vi "输入数据解析.vi"(0 "单个参数补充":dbl, 1 "从板号":dbl=1.0, 2 "主板二维码":string="BNET01", 3 "从板二维码":string="BNET01", 5 "主板引用":refnum<vi>, 7 "从板引用":refnum<vi>, 9 "主板选项":string="三级故障阀值", 11 "枚举":enum16{"主板", "从板"}(ring), 12 "快换":bool caption="快换写入") -> (4 "输出数组":dbl[][](array[numeric]), 6 "数组长度":dbl[](array[numeric]), 8 "循环次数":i32, 10 "命令":u32, 14 "名称":string[](array[string]), 15 "命令序号":u32[](array[numeric]))   [LabVIEW 2013] (continued)
                  disable-tunnel: [w17680 w17684] -> w17676
                  disable-tunnel: w17674 -> [w17679 _]
                  frame Disabled {
                    n6928 = Unbundle By Name(w17679) -> ("电压过高"=w17678:dbl)
                    n6929 = call "输入分辨率计算-EV05.vi"("1字节?"=FALSE, "数值"=w17678, "分辨率"=0.1) -> ("低字节"=w17680:dbl, "高字节1"=w17681:dbl)  [unwired: 2 in, 5 out]
                  }
                  frame Enabled {
                    w17684 = 255 ("高字节1")
                  }
                }
                n6930 = Build Array(w17677, w17676) -> (w17675:i32[])
              }
              frame 1 {
                # "电压过低"
                n6931 = disable-structure shown="启用" {
                  disable-tunnel: [w17692 w17695] -> w17688
                  disable-tunnel: [w17691 w17695] -> w17687
                  disable-tunnel: w17685 -> [w17690 _]
                  frame Disabled {
                    n6932 = Unbundle By Name(w17690) -> ("电压过低"=w17689:dbl)
                    n6933 = call "输入分辨率计算-EV05.vi"("1字节?"=FALSE, "数值"=w17689, "分辨率"=0.1) -> ("低字节"=w17691:dbl, "高字节1"=w17692:dbl)  [unwired: 2 in, 5 out]
                  }
                  frame Enabled {
                    w17695 = 255 ("高字节1")
                  }
                }
                n6934 = Build Array(w17688, w17687) -> (w17686:i32[])
              }
              frame 2 {
                # "电压不均衡"
                n6935 = disable-structure shown="启用" {
                  disable-tunnel: [w17703 w17706] -> w17699
                  disable-tunnel: [w17702 w17706] -> w17698
                  disable-tunnel: w17696 -> [w17701 _]
                  frame Disabled {
                    n6936 = Unbundle By Name(w17701) -> ("电压不均衡(V)"=w17700:dbl)
                    n6937 = call "输入分辨率计算-EV05.vi"("1字节?"=FALSE, "数值"=w17700, "分辨率"=0.1) -> ("低字节"=w17702:dbl, "高字节1"=w17703:dbl)  [unwired: 2 in, 5 out]
                  }
                  frame Enabled {
                    w17706 = 255 ("高字节1")
                  }
                }
                n6938 = Build Array(w17699, w17698) -> (w17697:i32[])
              }
              frame 3 {
                # "温度过高"
                n6939 = disable-structure shown="启用" {
                  disable-tunnel: [w17713 255 ("高字节1")] -> w17709
                  disable-tunnel: w17707 -> [w17711 _]
                  frame Enabled {
                    n6940 = Unbundle By Name(w17711) -> ("温度过高"=w17710:dbl)
                    n6941 = call "输入分辨率计算-EV05.vi"("1字节?"=TRUE, "数值"=w17710, "偏移量"=-40.0, "分辨率"=1.0) -> ("高字节1"=w17713:dbl)  [unwired: 1 in, 6 out]
                  }
                  frame Disabled {
                  }
                }
                n6942 = Build Array(w17709) -> (w17708:dbl[])
              }
              frame 4 {
                # "温度过低"
                n6943 = disable-structure shown="启用" {
                  disable-tunnel: [w17723 255 ("高字节1")] -> w17719
                  disable-tunnel: w17717 -> [w17721 _]
                  frame Disabled {
                    n6944 = Unbundle By Name(w17721) -> ("温度过低"=w17720:dbl)
                    n6945 = call "输入分辨率计算-EV05.vi"("1字节?"=TRUE, "数值"=w17720, "偏移量"=-40.0, "分辨率"=1.0) -> ("高字节1"=w17723:dbl)  [unwired: 1 in, 6 out]
                  }
                  frame Enabled {
                  }
                }
                n6946 = Build Array(w17719) -> (w17718:i32[])
              }
              frame 5 {
                # "温度不均衡"
                n6947 = disable-structure shown="启用" {
                  disable-tunnel: [w17732 255 ("高字节1")] -> w17729
                  disable-tunnel: w17727 -> [w17731 _]
                  frame Disabled {
                    n6948 = Unbundle By Name(w17731) -> ("温度不均衡"=w17730:dbl)
                    n6949 = call "输入分辨率计算-EV05.vi"("1字节?"=TRUE, "数值"=w17730, "分辨率"=1.0) -> ("高字节1"=w17732:dbl)  [unwired: 2 in, 6 out]
                  }
                  frame Enabled {
                  }
                }
                n6950 = Build Array(w17729) -> (w17728:i32[])
              }
              frame 6 {
                # "SOC过低"
                n6951 = disable-structure shown="启用" {
                  disable-tunnel: w17738 -> [w17755 _]
                  disable-tunnel: [w17741 w17758] -> w17737
                  disable-tunnel: [w17740 w17758] -> w17736
                  frame Disabled {
                    n6952 = Unbundle By Name(w17755) -> ("SOC过低"=w17754:dbl)
                    n6953 = call "输入分辨率计算-EV05.vi"("1字节?"=FALSE, "数值"=w17754, "分辨率"=0.1) -> ("低字节"=w17743:dbl, "高字节1"=w17744:dbl)  [unwired: 2 in, 5 out]
                    n6954 = call "二进制解析-8.6.vi"("索引"=4, "数值"=0) -> ("低位子数组"=w17747:i32[])  [unwired: 3 out]
                    n6955 = call "二进制解析-8.6.vi"("索引"=4, "数值"=w17744) -> ("低位子数组"=w17750:i32[])  [unwired: 3 out]
                    n6956 = call "二进制解析-8.6.vi"("索引"=4, "数值"=w17743) -> ("低位子数组"=w17748:i32[], "高位子数组"=w17749:i32[])  [unwired: 2 out]
                    n6957 = Insert Into Array(array=w17750, new element=w17749) -> (w17752:i32[])  [unwired: 1 in]
                    n6958 = Insert Into Array(array=w17748, new element=w17747) -> (w17746:i32[])  [unwired: 1 in]
                    n6959 = call "数值二进制转十进制-8.6.vi"("子数组"=w17746) -> ("十进制数值"=w17741:i32)  [unwired: 4 out]
                    n6960 = call "数值二进制转十进制-8.6.vi"("子数组"=w17752) -> ("十进制数值"=w17740:i32)  [unwired: 4 out]
                  }
                  frame Enabled {
                    w17758 = 255 ("高字节1")
                  }
                }
                n6961 = Build Array(w17736, w17737) -> (w17739:i32[])
              }
            }
            n6962 = Insert Into Array(array=w17670, new element=w17669) -> (w17671:dbl[])  [unwired: 1 in]
          }
          n6963 = Build Array(w17664) -> (w17663:dbl[][])
        }
        frame "温度过高(3)" {
          n6964 = Unbundle By Name(w17763) -> ("三级故障(从板)"=w17764:refnum<vi>)
          n6965 = property class="Clust (严格)"(reference=w17764) -> ("Value"=w17762:T8)  [unwired: 1 in, 2 out]
          n6966 = for {
            N: 7 -> [_]
            tunnel: w17762 -> [w17774]
            shift-right: [w17773] -> w17766
            shift-left: dbl[] [] -> [w17772]
            i -> [w17775]
            n6967 = case shown="3" w17775 {
              tunnel: w17774 -> [w17776 w17787 w17798 w17809 w17819 w17829 w17840]
              tunnel: [w17777 w17788 w17799 w17810 w17820 w17830 w17841] -> w17771
              frame 0, Default {
                # "电压过高"
                n6968 = disable-structure shown="启用" {
                  disable-tunnel: [w17783 w17786] -> w17779
                  disable-tunnel: [w17782 w17786] -> w17778
                  disable-tunnel: w17776 -> [w17781 _]
                  frame Disabled {
                    n6969 = Unbundle By Name(w17781) -> ("电压过高"=w17780:dbl)
                    n6970 = call "输入分辨率计算-EV05.vi"("1字节?"=FALSE, "数值"=w17780, "分辨率"=0.1) -> ("低字节"=w17782:dbl, "高字节1"=w17783:dbl)  [unwired: 2 in, 5 out]
                  }
                  frame Enabled {
                    w17786 = 255 ("高字节1")
                  }
                }
                n6971 = Build Array(w17779, w17778) -> (w17777:i32[])
              }
              frame 1 {
                # "电压过低"
                n6972 = disable-structure shown="启用" {
                  disable-tunnel: [w17794 w17797] -> w17790
                  disable-tunnel: [w17793 w17797] -> w17789
                  disable-tunnel: w17787 -> [w17792 _]
                  frame Disabled {
                    n6973 = Unbundle By Name(w17792) -> ("电压过低"=w17791:dbl)
                    n6974 = call "输入分辨率计算-EV05.vi"("1字节?"=FALSE, "数值"=w17791, "分辨率"=0.1) -> ("低字节"=w17793:dbl, "高字节1"=w17794:dbl)  [unwired: 2 in, 5 out]
                  }
                  frame Enabled {
                    w17797 = 255 ("高字节1")
                  }
                }
                n6975 = Build Array(w17790, w17789) -> (w17788:i32[])
              }
              frame 2 {
                # "电压不均衡"
                n6976 = disable-structure shown="启用" {
                  disable-tunnel: [w17805 w17808] -> w17801
                  disable-tunnel: [w17804 w17808] -> w17800
                  disable-tunnel: w17798 -> [w17803 _]
                  frame Disabled {
                    n6977 = Unbundle By Name(w17803) -> ("电压不均衡(V)"=w17802:dbl)
                    n6978 = call "输入分辨率计算-EV05.vi"("1字节?"=FALSE, "数值"=w17802, "分辨率"=0.1) -> ("低字节"=w17804:dbl, "高字节1"=w17805:dbl)  [unwired: 2 in, 5 out]
                  }
                  frame Enabled {
                    w17808 = 255 ("高字节1")
                  }
                }
                n6979 = Build Array(w17801, w17800) -> (w17799:i32[])
              }
              frame 3 {
                # "温度过高"
                n6980 = disable-structure shown="启用" {
                  disable-tunnel: [w17815 255 ("高字节1")] -> w17811
                  disable-tunnel: w17809 -> [w17813 _]
                  frame Enabled {
                    n6981 = Unbundle By Name(w17813) -> ("温度过高"=w17812:dbl)
                    n6982 = call "输入分辨率计算-EV05.vi"("1字节?"=TRUE, "数值"=w17812, "偏移量"=-40.0, "分辨率"=1.0) -> ("高字节1"=w17815:dbl)  [unwired: 1 in, 6 out]
                  }
                  frame Disabled {
                  }
                }
                n6983 = Build Array(w17811) -> (w17810:dbl[])
              }
              frame 4 {
                # "温度过低"
                n6984 = disable-structure shown="启用" {
                  disable-tunnel: [w17825 255 ("高字节1")] -> w17821
                  disable-tunnel: w17819 -> [w17823 _]
                  frame Disabled {
                    n6985 = Unbundle By Name(w17823) -> ("温度过低"=w17822:dbl)
                    n6986 = call "输入分辨率计算-EV05.vi"("1字节?"=TRUE, "数值"=w17822, "偏移量"=-40.0, "分辨率"=1.0) -> ("高字节1"=w17825:dbl)  [unwired: 1 in, 6 out]
                  }
                  frame Enabled {
                  }
                }
                n6987 = Build Array(w17821) -> (w17820:i32[])
              }
              frame 5 {
                # "温度不均衡"
                n6988 = disable-structure shown="启用" {
                  disable-tunnel: [w17834 255 ("高字节1")] -> w17831
                  disable-tunnel: w17829 -> [w17833 _]
                  frame Disabled {
                    n6989 = Unbundle By Name(w17833) -> ("温度不均衡"=w17832:dbl)
                    n6990 = call "输入分辨率计算-EV05.vi"("1字节?"=TRUE, "数值"=w17832, "分辨率"=1.0) -> ("高字节1"=w17834:dbl)  [unwired: 2 in, 6 out]
                  }
                  frame Enabled {
                  }
                }
                n6991 = Build Array(w17831) -> (w17830:i32[])
              }
              frame 6 {
                # "SOC过低"
                n6992 = disable-structure shown="启用" {
                  disable-tunnel: w17840 -> [w17857 _]
                  disable-tunnel: [w17843 w17860] -> w17839
                  disable-tunnel: [w17842 w17860] -> w17838
                  frame Disabled {
                    n6993 = Unbundle By Name(w17857) -> ("SOC过低"=w17856:dbl)
                    n6994 = call "输入分辨率计算-EV05.vi"("1字节?"=FALSE, "数值"=w17856, "分辨率"=0.1) -> ("低字节"=w17845:dbl, "高字节1"=w17846:dbl)  [unwired: 2 in, 5 out]
                    n6995 = call "二进制解析-8.6.vi"("索引"=4, "数值"=0) -> ("低位子数组"=w17849:i32[])  [unwired: 3 out]
                    n6996 = call "二进制解析-8.6.vi"("索引"=4, "数值"=w17846) -> ("低位子数组"=w17852:i32[])  [unwired: 3 out]
                    n6997 = call "二进制解析-8.6.vi"("索引"=4, "数值"=w17845) -> ("低位子数组"=w17850:i32[], "高位子数组"=w17851:i32[])  [unwired: 2 out]
                    n6998 = Insert Into Array(array=w17852, new element=w17851) -> (w17854:i32[])  [unwired: 1 in]
                    n6999 = Insert Into Array(array=w17850, new element=w17849) -> (w17848:i32[])  [unwired: 1 in]
                    n7000 = call "数值二进制转十进制-8.6.vi"("子数组"=w17848) -> ("十进制数值"=w17843:i32)  [unwired: 4 out]
                    n7001 = call "数值二进制转十进制-8.6.vi"("子数组"=w17854) -> ("十进制数值"=w17842:i32)  [unwired: 4 out]
                  }
                  frame Enabled {
                    w17860 = 255 ("高字节1")
                  }
                }
                n7002 = Build Array(w17838, w17839) -> (w17841:i32[])
              }
            }
            n7003 = Insert Into Array(array=w17772, new element=w17771) -> (w17773:dbl[])  [unwired: 1 in]
          }
          n7004 = Build Array(w17766) -> (w17765:dbl[][])
        }
        frame "温度过低" {
          n7005 = Unbundle By Name(w17865) -> ("一级故障(从板)"=w17866:refnum<vi>)
          n7006 = property class="Clust (严格)"(reference=w17866) -> ("Value"=w17864:T8)  [unwired: 1 in, 2 out]
          n7007 = for {
            N: 7 -> [_]
            tunnel: w17864 -> [w17876]
            shift-right: [w17875] -> w17868
            shift-left: dbl[] [] -> [w17874]
            i -> [w17877]
            n7008 = case shown="4" w17877 {
              tunnel: w17876 -> [w17878 w17889 w17900 w17911 w17921 w17931 w17942]
              tunnel: [w17879 w17890 w17901 w17912 w17922 w17932 w17943] -> w17873
              frame 0, Default {
                # "电压过高"
                n7009 = disable-structure shown="启用" {
                  disable-tunnel: [w17885 w17888] -> w17881
                  disable-tunnel: [w17884 w17888] -> w17880
                  disable-tunnel: w17878 -> [w17883 _]
                  frame Disabled {
                    n7010 = Unbundle By Name(w17883) -> ("电压过高"=w17882:dbl)
                    n7011 = call "输入分辨率计算-EV05.vi"("1字节?"=FALSE, "数值"=w17882, "分辨率"=0.1) -> ("低字节"=w17884:dbl, "高字节1"=w17885:dbl)  [unwired: 2 in, 5 out]
                  }
                  frame Enabled {
                    w17888 = 255 ("高字节1")
                  }
                }
                n7012 = Build Array(w17881, w17880) -> (w17879:i32[])
              }
              frame 1 {
                # "电压过低"
                n7013 = disable-structure shown="启用" {
                  disable-tunnel: [w17896 w17899] -> w17892
                  disable-tunnel: [w17895 w17899] -> w17891
                  disable-tunnel: w17889 -> [w17894 _]
                  frame Disabled {
                    n7014 = Unbundle By Name(w17894) -> ("电压过低"=w17893:dbl)
                    n7015 = call "输入分辨率计算-EV05.vi"("1字节?"=FALSE, "数值"=w17893, "分辨率"=0.1) -> ("低字节"=w17895:dbl, "高字节1"=w17896:dbl)  [unwired: 2 in, 5 out]
                  }
                  frame Enabled {
                    w17899 = 255 ("高字节1")
                  }
                }
                n7016 = Build Array(w17892, w17891) -> (w17890:i32[])
              }
              frame 2 {
                # "电压不均衡"
                n7017 = disable-structure shown="启用" {
                  disable-tunnel: [w17907 w17910] -> w17903
                  disable-tunnel: [w17906 w17910] -> w17902
                  disable-tunnel: w17900 -> [w17905 _]
                  frame Disabled {
                    n7018 = Unbundle By Name(w17905) -> ("电压不均衡(V)"=w17904:dbl)
                    n7019 = call "输入分辨率计算-EV05.vi"("1字节?"=FALSE, "数值"=w17904, "分辨率"=0.1) -> ("低字节"=w17906:dbl, "高字节1"=w17907:dbl)  [unwired: 2 in, 5 out]
                  }
                  frame Enabled {
                    w17910 = 255 ("高字节1")
                  }
                }
                n7020 = Build Array(w17903, w17902) -> (w17901:i32[])
              }
              frame 3 {
                # "温度过高"
                n7021 = disable-structure shown="启用" {
                  disable-tunnel: [w17917 255 ("高字节1")] -> w17913
                  disable-tunnel: w17911 -> [w17915 _]
                  frame Disabled {
                    n7022 = Unbundle By Name(w17915) -> ("温度过高"=w17914:dbl)
                    n7023 = call "输入分辨率计算-EV05.vi"("1字节?"=TRUE, "数值"=w17914, "偏移量"=-40.0, "分辨率"=1.0) -> ("高字节1"=w17917:dbl)  [unwired: 1 in, 6 out]
                  }
                  frame Enabled {
                  }
                }
                n7024 = Build Array(w17913) -> (w17912:i32[])
              }
              frame 4 {
                # "温度过低"
                n7025 = disable-structure shown="启用" {
                  disable-tunnel: [w17927 255 ("高字节1")] -> w17923
                  disable-tunnel: w17921 -> [w17925 _]
                  frame Enabled {
                    n7026 = Unbundle By Name(w17925) -> ("温度过低"=w17924:dbl)
                    n7027 = call "输入分辨率计算-EV05.vi"("1字节?"=TRUE, "数值"=w17924, "偏移量"=-40.0, "分辨率"=1.0) -> ("高字节1"=w17927:dbl)  [unwired: 1 in, 6 out]
                  }
                  frame Disabled {
                  }
                }
                n7028 = Build Array(w17923) -> (w17922:dbl[])
              }
              frame 5 {
                # "温度不均衡"
                n7029 = disable-structure shown="启用" {
                  disable-tunnel: [w17936 255 ("高字节1")] -> w17933
                  disable-tunnel: w17931 -> [w17935 _]
                  frame Disabled {
                    n7030 = Unbundle By Name(w17935) -> ("温度不均衡"=w17934:dbl)
                    n7031 = call "输入分辨率计算-EV05.vi"("1字节?"=TRUE, "数值"=w17934, "分辨率"=1.0) -> ("高字节1"=w17936:dbl)  [unwired: 2 in, 6 out]
                  }
                  frame Enabled {
                  }
                }
                n7032 = Build Array(w17933) -> (w17932:i32[])
              }
              frame 6 {
                # "SOC过低"
                n7033 = disable-structure shown="启用" {
                  disable-tunnel: w17942 -> [w17959 _]
                  disable-tunnel: [w17945 w17962] -> w17941
                  disable-tunnel: [w17944 w17962] -> w17940
                  frame Disabled {
                    n7034 = Unbundle By Name(w17959) -> ("SOC过低"=w17958:dbl)
                    n7035 = call "输入分辨率计算-EV05.vi"("1字节?"=FALSE, "数值"=w17958, "分辨率"=0.1) -> ("低字节"=w17947:dbl, "高字节1"=w17948:dbl)  [unwired: 2 in, 5 out]
                    n7036 = call "二进制解析-8.6.vi"("索引"=4, "数值"=0) -> ("低位子数组"=w17951:i32[])  [unwired: 3 out]
                    n7037 = call "二进制解析-8.6.vi"("索引"=4, "数值"=w17948) -> ("低位子数组"=w17954:i32[])  [unwired: 3 out]
                    n7038 = call "二进制解析-8.6.vi"("索引"=4, "数值"=w17947) -> ("低位子数组"=w17952:i32[], "高位子数组"=w17953:i32[])  [unwired: 2 out]
                    n7039 = Insert Into Array(array=w17954, new element=w17953) -> (w17956:i32[])  [unwired: 1 in]
                    n7040 = Insert Into Array(array=w17952, new element=w17951) -> (w17950:i32[])  [unwired: 1 in]
                    n7041 = call "数值二进制转十进制-8.6.vi"("子数组"=w17950) -> ("十进制数值"=w17945:i32)  [unwired: 4 out]
                    n7042 = call "数值二进制转十进制-8.6.vi"("子数组"=w17956) -> ("十进制数值"=w17944:i32)  [unwired: 4 out]
                  }
                  frame Enabled {
                    w17962 = 255 ("高字节1")
                  }
                }
                n7043 = Build Array(w17940, w17941) -> (w17943:i32[])
              }
            }
            n7044 = Insert Into Array(array=w17874, new element=w17873) -> (w17875:dbl[])  [unwired: 1 in]
          }
          n7045 = Build Array(w17868) -> (w17867:dbl[][])
        }
        frame "温度过低(2)" {
          n7046 = Unbundle By Name(w17967) -> ("二级故障(从板)"=w17968:refnum<vi>)
          n7047 = property class="Clust (严格)"(reference=w17968) -> ("Value"=w17966:T8)  [unwired: 1 in, 2 out]
          n7048 = for {
            N: 7 -> [_]
            tunnel: w17966 -> [w17978]
            shift-right: [w17977] -> w17970
            shift-left: dbl[] [] -> [w17976]
            i -> [w17979]
            n7049 = case shown="4" w17979 {
              tunnel: w17978 -> [w17980 w17991 w18002 w18013 w18023 w18033 w18044]
              tunnel: [w17981 w17992 w18003 w18014 w18024 w18034 w18045] -> w17975
              frame 0, Default {
                # "电压过高"
                n7050 = disable-structure shown="启用" {
                  disable-tunnel: [w17987 w17990] -> w17983
                  disable-tunnel: [w17986 w17990] -> w17982
                  disable-tunnel: w17980 -> [w17985 _]
                  frame Disabled {
                    n7051 = Unbundle By Name(w17985) -> ("电压过高"=w17984:dbl)
                    n7052 = call "输入分辨率计算-EV05.vi"("1字节?"=FALSE, "数值"=w17984, "分辨率"=0.1) -> ("低字节"=w17986:dbl, "高字节1"=w17987:dbl)  [unwired: 2 in, 5 out]
                  }
                  frame Enabled {
                    w17990 = 255 ("高字节1")
                  }
                }
                n7053 = Build Array(w17983, w17982) -> (w17981:i32[])
              }
              frame 1 {
                # "电压过低"
                n7054 = disable-structure shown="启用" {
                  disable-tunnel: [w17998 w18001] -> w17994
                  disable-tunnel: [w17997 w18001] -> w17993
                  disable-tunnel: w17991 -> [w17996 _]
                  frame Disabled {
                    n7055 = Unbundle By Name(w17996) -> ("电压过低"=w17995:dbl)
                    n7056 = call "输入分辨率计算-EV05.vi"("1字节?"=FALSE, "数值"=w17995, "分辨率"=0.1) -> ("低字节"=w17997:dbl, "高字节1"=w17998:dbl)  [unwired: 2 in, 5 out]
                  }
                  frame Enabled {
                    w18001 = 255 ("高字节1")
                  }
                }
                n7057 = Build Array(w17994, w17993) -> (w17992:i32[])
              }
              frame 2 {
                # "电压不均衡"
                n7058 = disable-structure shown="启用" {
                  disable-tunnel: [w18009 w18012] -> w18005
                  disable-tunnel: [w18008 w18012] -> w18004
                  disable-tunnel: w18002 -> [w18007 _]
                  frame Disabled {
                    n7059 = Unbundle By Name(w18007) -> ("电压不均衡(V)"=w18006:dbl)
                    n7060 = call "输入分辨率计算-EV05.vi"("1字节?"=FALSE, "数值"=w18006, "分辨率"=0.1) -> ("低字节"=w18008:dbl, "高字节1"=w18009:dbl)  [unwired: 2 in, 5 out]
                  }
                  frame Enabled {
                    w18012 = 255 ("高字节1")
                  }
                }
                n7061 = Build Array(w18005, w18004) -> (w18003:i32[])
              }
              frame 3 {
                # "温度过高"
                n7062 = disable-structure shown="启用" {
                  disable-tunnel: [w18019 255 ("高字节1")] -> w18015
                  disable-tunnel: w18013 -> [w18017 _]
                  frame Disabled {
                    n7063 = Unbundle By Name(w18017) -> ("温度过高"=w18016:dbl)
                    n7064 = call "输入分辨率计算-EV05.vi"("1字节?"=TRUE, "数值"=w18016, "偏移量"=-40.0, "分辨率"=1.0) -> ("高字节1"=w18019:dbl)  [unwired: 1 in, 6 out]
                  }
                  frame Enabled {
                  }
                }
                n7065 = Build Array(w18015) -> (w18014:i32[])
              }
              frame 4 {
                # "温度过低"
                n7066 = disable-structure shown="启用" {
                  disable-tunnel: [w18029 255 ("高字节1")] -> w18025
                  disable-tunnel: w18023 -> [w18027 _]
                  frame Enabled {
                    n7067 = Unbundle By Name(w18027) -> ("温度过低"=w18026:dbl)
                    n7068 = call "输入分辨率计算-EV05.vi"("1字节?"=TRUE, "数值"=w18026, "偏移量"=-40.0, "分辨率"=1.0) -> ("高字节1"=w18029:dbl)  [unwired: 1 in, 6 out]
                  }
                  frame Disabled {
                  }
                }
                n7069 = Build Array(w18025) -> (w18024:dbl[])
              }
              frame 5 {
                # "温度不均衡"
                n7070 = disable-structure shown="启用" {
                  disable-tunnel: [w18038 255 ("高字节1")] -> w18035
                  disable-tunnel: w18033 -> [w18037 _]
                  frame Disabled {
                    n7071 = Unbundle By Name(w18037) -> ("温度不均衡"=w18036:dbl)
                    n7072 = call "输入分辨率计算-EV05.vi"("1字节?"=TRUE, "数值"=w18036, "分辨率"=1.0) -> ("高字节1"=w18038:dbl)  [unwired: 2 in, 6 out]
                  }
                  frame Enabled {
                  }
                }
                n7073 = Build Array(w18035) -> (w18034:i32[])
              }
              frame 6 {
                # "SOC过低"
                n7074 = disable-structure shown="启用" {
                  disable-tunnel: w18044 -> [w18061 _]
                  disable-tunnel: [w18047 w18064] -> w18043
                  disable-tunnel: [w18046 w18064] -> w18042
                  frame Disabled {
                    n7075 = Unbundle By Name(w18061) -> ("SOC过低"=w18060:dbl)
                    n7076 = call "输入分辨率计算-EV05.vi"("1字节?"=FALSE, "数值"=w18060, "分辨率"=0.1) -> ("低字节"=w18049:dbl, "高字节1"=w18050:dbl)  [unwired: 2 in, 5 out]
                    n7077 = call "二进制解析-8.6.vi"("索引"=4, "数值"=0) -> ("低位子数组"=w18053:i32[])  [unwired: 3 out]
                    n7078 = call "二进制解析-8.6.vi"("索引"=4, "数值"=w18050) -> ("低位子数组"=w18056:i32[])  [unwired: 3 out]
                    n7079 = call "二进制解析-8.6.vi"("索引"=4, "数值"=w18049) -> ("低位子数组"=w18054:i32[], "高位子数组"=w18055:i32[])  [unwired: 2 out]
                    n7080 = Insert Into Array(array=w18056, new element=w18055) -> (w18058:i32[])  [unwired: 1 in]
                    n7081 = Insert Into Array(array=w18054, new element=w18053) -> (w18052:i32[])  [unwired: 1 in]
                    n7082 = call "数值二进制转十进制-8.6.vi"("子数组"=w18052) -> ("十进制数值"=w18047:i32)  [unwired: 4 out]
                    n7083 = call "数值二进制转十进制-8.6.vi"("子数组"=w18058) -> ("十进制数值"=w18046:i32)  [unwired: 4 out]
                  }
                  frame Enabled {
                    w18064 = 255 ("高字节1")
                  }
                }
                n7084 = Build Array(w18042, w18043) -> (w18045:i32[])
              }
            }
            n7085 = Insert Into Array(array=w17976, new element=w17975) -> (w17977:dbl[])  [unwired: 1 in]
          }
          n7086 = Build Array(w17970) -> (w17969:dbl[][])
        }
        frame "温度过低(3)" {
          n7087 = Unbundle By Name(w18069) -> ("三级故障(从板)"=w18070:refnum<vi>)
          n7088 = property class="Clust (严格)"(reference=w18070) -> ("Value"=w18068:T8)  [unwired: 1 in, 2 out]
          n7089 = for {
            N: 7 -> [_]
            tunnel: w18068 -> [w18080]
            shift-right: [w18079] -> w18072
            shift-left: dbl[] [] -> [w18078]
            i -> [w18081]
            n7090 = case shown="4" w18081 {
              tunnel: w18080 -> [w18082 w18093 w18104 w18115 w18125 w18135 w18146]
              tunnel: [w18083 w18094 w18105 w18116 w18126 w18136 w18147] -> w18077
              frame 0, Default {
                # "电压过高"
                n7091 = disable-structure shown="启用" {
                  disable-tunnel: [w18089 w18092] -> w18085
                  disable-tunnel: [w18088 w18092] -> w18084
                  disable-tunnel: w18082 -> [w18087 _]
                  frame Disabled {
                    n7092 = Unbundle By Name(w18087) -> ("电压过高"=w18086:dbl)
                    n7093 = call "输入分辨率计算-EV05.vi"("1字节?"=FALSE, "数值"=w18086, "分辨率"=0.1) -> ("低字节"=w18088:dbl, "高字节1"=w18089:dbl)  [unwired: 2 in, 5 out]
                  }
                  frame Enabled {
                    w18092 = 255 ("高字节1")
                  }
                }
                n7094 = Build Array(w18085, w18084) -> (w18083:i32[])
              }
              frame 1 {
                # "电压过低"
                n7095 = disable-structure shown="启用" {
                  disable-tunnel: [w18100 w18103] -> w18096
                  disable-tunnel: [w18099 w18103] -> w18095
                  disable-tunnel: w18093 -> [w18098 _]
                  frame Disabled {
                    n7096 = Unbundle By Name(w18098) -> ("电压过低"=w18097:dbl)
                    n7097 = call "输入分辨率计算-EV05.vi"("1字节?"=FALSE, "数值"=w18097, "分辨率"=0.1) -> ("低字节"=w18099:dbl, "高字节1"=w18100:dbl)  [unwired: 2 in, 5 out]
                  }
                  frame Enabled {
                    w18103 = 255 ("高字节1")
                  }
                }
                n7098 = Build Array(w18096, w18095) -> (w18094:i32[])
              }
              frame 2 {
                # "电压不均衡"
                n7099 = disable-structure shown="启用" {
                  disable-tunnel: [w18111 w18114] -> w18107
                  disable-tunnel: [w18110 w18114] -> w18106
                  disable-tunnel: w18104 -> [w18109 _]
                  frame Disabled {
                    n7100 = Unbundle By Name(w18109) -> ("电压不均衡(V)"=w18108:dbl)
                    n7101 = call "输入分辨率计算-EV05.vi"("1字节?"=FALSE, "数值"=w18108, "分辨率"=0.1) -> ("低字节"=w18110:dbl, "高字节1"=w18111:dbl)  [unwired: 2 in, 5 out]
                  }
                  frame Enabled {
                    w18114 = 255 ("高字节1")
                  }
                }
                n7102 = Build Array(w18107, w18106) -> (w18105:i32[])
              }
              frame 3 {
                # "温度过高"
                n7103 = disable-structure shown="启用" {
                  disable-tunnel: [w18121 255 ("高字节1")] -> w18117
                  disable-tunnel: w18115 -> [w18119 _]
                  frame Disabled {
                    n7104 = Unbundle By Name(w18119) -> ("温度过高"=w18118:dbl)
                    n7105 = call "输入分辨率计算-EV05.vi"("1字节?"=TRUE, "数值"=w18118, "偏移量"=-40.0, "分辨率"=1.0) -> ("高字节1"=w18121:dbl)  [unwired: 1 in, 6 out]
                  }
                  frame Enabled {
                  }
                }
                n7106 = Build Array(w18117) -> (w18116:i32[])
              }
              frame 4 {
                # "温度过低"
                n7107 = disable-structure shown="启用" {
                  disable-tunnel: [w18131 255 ("高字节1")] -> w18127
                  disable-tunnel: w18125 -> [w18129 _]
                  frame Enabled {
                    n7108 = Unbundle By Name(w18129) -> ("温度过低"=w18128:dbl)
                    n7109 = call "输入分辨率计算-EV05.vi"("1字节?"=TRUE, "数值"=w18128, "偏移量"=-40.0, "分辨率"=1.0) -> ("高字节1"=w18131:dbl)  [unwired: 1 in, 6 out]
                  }
                  frame Disabled {
                  }
                }
                n7110 = Build Array(w18127) -> (w18126:dbl[])
              }
              frame 5 {
                # "温度不均衡"
                n7111 = disable-structure shown="启用" {
                  disable-tunnel: [w18140 255 ("高字节1")] -> w18137
                  disable-tunnel: w18135 -> [w18139 _]
                  frame Disabled {
                    n7112 = Unbundle By Name(w18139) -> ("温度不均衡"=w18138:dbl)
                    n7113 = call "输入分辨率计算-EV05.vi"("1字节?"=TRUE, "数值"=w18138, "分辨率"=1.0) -> ("高字节1"=w18140:dbl)  [unwired: 2 in, 6 out]
                  }
                  frame Enabled {
                  }
                }
                n7114 = Build Array(w18137) -> (w18136:i32[])
              }
              frame 6 {
                # "SOC过低"
                n7115 = disable-structure shown="启用" {
                  disable-tunnel: w18146 -> [w18163 _]
                  disable-tunnel: [w18149 w18166] -> w18145
                  disable-tunnel: [w18148 w18166] -> w18144
                  frame Disabled {
                    n7116 = Unbundle By Name(w18163) -> ("SOC过低"=w18162:dbl)
                    n7117 = call "输入分辨率计算-EV05.vi"("1字节?"=FALSE, "数值"=w18162, "分辨率"=0.1) -> ("低字节"=w18151:dbl, "高字节1"=w18152:dbl)  [unwired: 2 in, 5 out]
                    n7118 = call "二进制解析-8.6.vi"("索引"=4, "数值"=0) -> ("低位子数组"=w18155:i32[])  [unwired: 3 out]
                    n7119 = call "二进制解析-8.6.vi"("索引"=4, "数值"=w18152) -> ("低位子数组"=w18158:i32[])  [unwired: 3 out]
                    n7120 = call "二进制解析-8.6.vi"("索引"=4, "数值"=w18151) -> ("低位子数组"=w18156:i32[], "高位子数组"=w18157:i32[])  [unwired: 2 out]
                    n7121 = Insert Into Array(array=w18158, new element=w18157) -> (w18160:i32[])  [unwired: 1 in]
                    n7122 = Insert Into Array(array=w18156, new element=w18155) -> (w18154:i32[])  [unwired: 1 in]
                    n7123 = call "数值二进制转十进制-8.6.vi"("子数组"=w18154) -> ("十进制数值"=w18149:i32)  [unwired: 4 out]
                    n7124 = call "数值二进制转十进制-8.6.vi"("子数组"=w18160) -> ("十进制数值"=w18148:i32)  [unwired: 4 out]
                  }
                  frame Enabled {
                    w18166 = 255 ("高字节1")
                  }
                }
                n7125 = Build Array(w18144, w18145) -> (w18147:i32[])
              }
            }
            n7126 = Insert Into Array(array=w18078, new element=w18077) -> (w18079:dbl[])  [unwired: 1 in]
          }
          n7127 = Build Array(w18072) -> (w18071:dbl[][])
        }
        frame "温度不均衡" {
          n7128 = Unbundle By Name(w18171) -> ("一级故障(从板)"=w18172:refnum<vi>)
          n7129 = property class="Clust (严格)"(reference=w18172) -> ("Value"=w18170:T8)  [unwired: 1 in, 2 out]
          n7130 = for {
            N: 7 -> [_]
            tunnel: w18170 -> [w18182]
            shift-right: [w18181] -> w18174
            shift-left: dbl[] [] -> [w18180]
            i -> [w18183]
            n7131 = case shown="5" w18183 {
              tunnel: w18182 -> [w18184 w18195 w18206 w18217 w18227 w18237 w18248]
              tunnel: [w18185 w18196 w18207 w18218 w18228 w18238 w18249] -> w18179
              frame 0, Default {
                # "电压过高"
                n7132 = disable-structure shown="启用" {
                  disable-tunnel: [w18191 w18194] -> w18187
                  disable-tunnel: [w18190 w18194] -> w18186
                  disable-tunnel: w18184 -> [w18189 _]
                  frame Disabled {
                    n7133 = Unbundle By Name(w18189) -> ("电压过高"=w18188:dbl)
                    n7134 = call "输入分辨率计算-EV05.vi"("1字节?"=FALSE, "数值"=w18188, "分辨率"=0.1) -> ("低字节"=w18190:dbl, "高字节1"=w18191:dbl)  [unwired: 2 in, 5 out]
                  }
                  frame Enabled {
                    w18194 = 255 ("高字节1")
                  }
                }
                n7135 = Build Array(w18187, w18186) -> (w18185:i32[])
              }
              frame 1 {
                # "电压过低"
                n7136 = disable-structure shown="启用" {
                  disable-tunnel: [w18202 w18205] -> w18198
                  disable-tunnel: [w18201 w18205] -> w18197
                  disable-tunnel: w18195 -> [w18200 _]
                  frame Disabled {
                    n7137 = Unbundle By Name(w18200) -> ("电压过低"=w18199:dbl)
                    n7138 = call "输入分辨率计算-EV05.vi"("1字节?"=FALSE, "数值"=w18199, "分辨率"=0.1) -> ("低字节"=w18201:dbl, "高字节1"=w18202:dbl)  [unwired: 2 in, 5 out]
                  }
                  frame Enabled {
                    w18205 = 255 ("高字节1")
                  }
                }
                n7139 = Build Array(w18198, w18197) -> (w18196:i32[])
              }
              frame 2 {
                # "电压不均衡"
                n7140 = disable-structure shown="启用" {
                  disable-tunnel: [w18213 w18216] -> w18209
                  disable-tunnel: [w18212 w18216] -> w18208
                  disable-tunnel: w18206 -> [w18211 _]
                  frame Disabled {
                    n7141 = Unbundle By Name(w18211) -> ("电压不均衡(V)"=w18210:dbl)
                    n7142 = call "输入分辨率计算-EV05.vi"("1字节?"=FALSE, "数值"=w18210, "分辨率"=0.1) -> ("低字节"=w18212:dbl, "高字节1"=w18213:dbl)  [unwired: 2 in, 5 out]
                  }
                  frame Enabled {
                    w18216 = 255 ("高字节1")
                  }
                }
                n7143 = Build Array(w18209, w18208) -> (w18207:i32[])
              }
              frame 3 {
                # "温度过高"
                n7144 = disable-structure shown="启用" {
                  disable-tunnel: [w18223 255 ("高字节1")] -> w18219
                  disable-tunnel: w18217 -> [w18221 _]
                  frame Disabled {
                    n7145 = Unbundle By Name(w18221) -> ("温度过高"=w18220:dbl)
                    n7146 = call "输入分辨率计算-EV05.vi"("1字节?"=TRUE, "数值"=w18220, "偏移量"=-40.0, "分辨率"=1.0) -> ("高字节1"=w18223:dbl)  [unwired: 1 in, 6 out]
                  }
                  frame Enabled {
                  }
                }
                n7147 = Build Array(w18219) -> (w18218:i32[])
              }
              frame 4 {
                # "温度过低"
                n7148 = disable-structure shown="启用" {
                  disable-tunnel: [w18233 255 ("高字节1")] -> w18229
                  disable-tunnel: w18227 -> [w18231 _]
                  frame Disabled {
                    n7149 = Unbundle By Name(w18231) -> ("温度过低"=w18230:dbl)
                    n7150 = call "输入分辨率计算-EV05.vi"("1字节?"=TRUE, "数值"=w18230, "偏移量"=-40.0, "分辨率"=1.0) -> ("高字节1"=w18233:dbl)  [unwired: 1 in, 6 out]
                  }
                  frame Enabled {
                  }
                }
                n7151 = Build Array(w18229) -> (w18228:i32[])
              }
              frame 5 {
                # "温度不均衡"
                n7152 = disable-structure shown="启用" {
                  disable-tunnel: [w18242 255 ("高字节1")] -> w18239
                  disable-tunnel: w18237 -> [w18241 _]
                  frame Enabled {
                    n7153 = Unbundle By Name(w18241) -> ("温度不均衡"=w18240:dbl)
                    n7154 = call "输入分辨率计算-EV05.vi"("1字节?"=TRUE, "数值"=w18240, "分辨率"=1.0) -> ("高字节1"=w18242:dbl)  [unwired: 2 in, 6 out]
                  }
                  frame Disabled {
                  }
                }
                n7155 = Build Array(w18239) -> (w18238:dbl[])
              }
              frame 6 {
                # "SOC过低"
                n7156 = disable-structure shown="启用" {
                  disable-tunnel: w18248 -> [w18265 _]
                  disable-tunnel: [w18251 w18268] -> w18247
                  disable-tunnel: [w18250 w18268] -> w18246
                  frame Disabled {
                    n7157 = Unbundle By Name(w18265) -> ("SOC过低"=w18264:dbl)
                    n7158 = call "输入分辨率计算-EV05.vi"("1字节?"=FALSE, "数值"=w18264, "分辨率"=0.1) -> ("低字节"=w18253:dbl, "高字节1"=w18254:dbl)  [unwired: 2 in, 5 out]
                    n7159 = call "二进制解析-8.6.vi"("索引"=4, "数值"=0) -> ("低位子数组"=w18257:i32[])  [unwired: 3 out]
                    n7160 = call "二进制解析-8.6.vi"("索引"=4, "数值"=w18254) -> ("低位子数组"=w18260:i32[])  [unwired: 3 out]
                    n7161 = call "二进制解析-8.6.vi"("索引"=4, "数值"=w18253) -> ("低位子数组"=w18258:i32[], "高位子数组"=w18259:i32[])  [unwired: 2 out]
                    n7162 = Insert Into Array(array=w18260, new element=w18259) -> (w18262:i32[])  [unwired: 1 in]
                    n7163 = Insert Into Array(array=w18258, new element=w18257) -> (w18256:i32[])  [unwired: 1 in]
                    n7164 = call "数值二进制转十进制-8.6.vi"("子数组"=w18256) -> ("十进制数值"=w18251:i32)  [unwired: 4 out]
                    n7165 = call "数值二进制转十进制-8.6.vi"("子数组"=w18262) -> ("十进制数值"=w18250:i32)  [unwired: 4 out]
                  }
                  frame Enabled {
                    w18268 = 255 ("高字节1")
                  }
                }
                n7166 = Build Array(w18246, w18247) -> (w18249:i32[])
              }
            }
            n7167 = Insert Into Array(array=w18180, new element=w18179) -> (w18181:dbl[])  [unwired: 1 in]
          }
          n7168 = Build Array(w18174) -> (w18173:dbl[][])
        }
        frame "温度不均衡(2)" {
          n7169 = Unbundle By Name(w18273) -> ("二级故障(从板)"=w18274:refnum<vi>)
          n7170 = property class="Clust (严格)"(reference=w18274) -> ("Value"=w18272:T8)  [unwired: 1 in, 2 out]
          n7171 = for {
            N: 7 -> [_]
            tunnel: w18272 -> [w18284]
            shift-right: [w18283] -> w18276
            shift-left: dbl[] [] -> [w18282]
            i -> [w18285]
            n7172 = case shown="5" w18285 {
              tunnel: w18284 -> [w18286 w18297 w18308 w18319 w18329 w18339 w18350]
              tunnel: [w18287 w18298 w18309 w18320 w18330 w18340 w18351] -> w18281
              frame 0, Default {
                # "电压过高"
                n7173 = disable-structure shown="启用" {
                  disable-tunnel: [w18293 w18296] -> w18289
                  disable-tunnel: [w18292 w18296] -> w18288
                  disable-tunnel: w18286 -> [w18291 _]
                  frame Disabled {
                    n7174 = Unbundle By Name(w18291) -> ("电压过高"=w18290:dbl)
                    n7175 = call "输入分辨率计算-EV05.vi"("1字节?"=FALSE, "数值"=w18290, "分辨率"=0.1) -> ("低字节"=w18292:dbl, "高字节1"=w18293:dbl)  [unwired: 2 in, 5 out]
                  }
                  frame Enabled {
                    w18296 = 255 ("高字节1")
                  }
                }
                n7176 = Build Array(w18289, w18288) -> (w18287:i32[])
              }
              frame 1 {
                # "电压过低"
                n7177 = disable-structure shown="启用" {
                  disable-tunnel: [w18304 w18307] -> w18300
                  disable-tunnel: [w18303 w18307] -> w18299
                  disable-tunnel: w18297 -> [w18302 _]
                  frame Disabled {
                    n7178 = Unbundle By Name(w18302) -> ("电压过低"=w18301:dbl)
                    n7179 = call "输入分辨率计算-EV05.vi"("1字节?"=FALSE, "数值"=w18301, "分辨率"=0.1) -> ("低字节"=w18303:dbl, "高字节1"=w18304:dbl)  [unwired: 2 in, 5 out]
                  }
                  frame Enabled {
                    w18307 = 255 ("高字节1")
                  }
                }
                n7180 = Build Array(w18300, w18299) -> (w18298:i32[])
              }
              frame 2 {
                # "电压不均衡"
                n7181 = disable-structure shown="启用" {
                  disable-tunnel: [w18315 w18318] -> w18311
                  disable-tunnel: [w18314 w18318] -> w18310
                  disable-tunnel: w18308 -> [w18313 _]
                  frame Disabled {
                    n7182 = Unbundle By Name(w18313) -> ("电压不均衡(V)"=w18312:dbl)
                    n7183 = call "输入分辨率计算-EV05.vi"("1字节?"=FALSE, "数值"=w18312, "分辨率"=0.1) -> ("低字节"=w18314:dbl, "高字节1"=w18315:dbl)  [unwired: 2 in, 5 out]
                  }
                  frame Enabled {
                    w18318 = 255 ("高字节1")
                  }
                }
                n7184 = Build Array(w18311, w18310) -> (w18309:i32[])
              }
              frame 3 {
                # "温度过高"
                n7185 = disable-structure shown="启用" {
                  disable-tunnel: [w18325 255 ("高字节1")] -> w18321
                  disable-tunnel: w18319 -> [w18323 _]
                  frame Disabled {
                    n7186 = Unbundle By Name(w18323) -> ("温度过高"=w18322:dbl)
                    n7187 = call "输入分辨率计算-EV05.vi"("1字节?"=TRUE, "数值"=w18322, "偏移量"=-40.0, "分辨率"=1.0) -> ("高字节1"=w18325:dbl)  [unwired: 1 in, 6 out]
                  }
                  frame Enabled {
                  }
                }
                n7188 = Build Array(w18321) -> (w18320:i32[])
              }
              frame 4 {
                # "温度过低"
                n7189 = disable-structure shown="启用" {
                  disable-tunnel: [w18335 255 ("高字节1")] -> w18331
                  disable-tunnel: w18329 -> [w18333 _]
                  frame Disabled {
                    n7190 = Unbundle By Name(w18333) -> ("温度过低"=w18332:dbl)
                    n7191 = call "输入分辨率计算-EV05.vi"("1字节?"=TRUE, "数值"=w18332, "偏移量"=-40.0, "分辨率"=1.0) -> ("高字节1"=w18335:dbl)  [unwired: 1 in, 6 out]
                  }
                  frame Enabled {
                  }
                }
                n7192 = Build Array(w18331) -> (w18330:i32[])
              }
              frame 5 {
                # "温度不均衡"
                n7193 = disable-structure shown="启用" {
                  disable-tunnel: [w18344 255 ("高字节1")] -> w18341
                  disable-tunnel: w18339 -> [w18343 _]
                  frame Enabled {
                    n7194 = Unbundle By Name(w18343) -> ("温度不均衡"=w18342:dbl)
                    n7195 = call "输入分辨率计算-EV05.vi"("1字节?"=TRUE, "数值"=w18342, "分辨率"=1.0) -> ("高字节1"=w18344:dbl)  [unwired: 2 in, 6 out]
                  }
                  frame Disabled {
                  }
                }
                n7196 = Build Array(w18341) -> (w18340:dbl[])
              }
              frame 6 {
                # "SOC过低"
                n7197 = disable-structure shown="启用" {
                  disable-tunnel: w18350 -> [w18367 _]
                  disable-tunnel: [w18353 w18370] -> w18349
                  disable-tunnel: [w18352 w18370] -> w18348
                  frame Disabled {
                    n7198 = Unbundle By Name(w18367) -> ("SOC过低"=w18366:dbl)
                    n7199 = call "输入分辨率计算-EV05.vi"("1字节?"=FALSE, "数值"=w18366, "分辨率"=0.1) -> ("低字节"=w18355:dbl, "高字节1"=w18356:dbl)  [unwired: 2 in, 5 out]
                    n7200 = call "二进制解析-8.6.vi"("索引"=4, "数值"=0) -> ("低位子数组"=w18359:i32[])  [unwired: 3 out]
                    n7201 = call "二进制解析-8.6.vi"("索引"=4, "数值"=w18356) -> ("低位子数组"=w18362:i32[])  [unwired: 3 out]
                    n7202 = call "二进制解析-8.6.vi"("索引"=4, "数值"=w18355) -> ("低位子数组"=w18360:i32[], "高位子数组"=w18361:i32[])  [unwired: 2 out]
                    n7203 = Insert Into Array(array=w18362, new element=w18361) -> (w18364:i32[])  [unwired: 1 in]
                    n7204 = Insert Into Array(array=w18360, new element=w18359) -> (w18358:i32[])  [unwired: 1 in]
                    n7205 = call "数值二进制转十进制-8.6.vi"("子数组"=w18358) -> ("十进制数值"=w18353:i32)  [unwired: 4 out]
                    n7206 = call "数值二进制转十进制-8.6.vi"("子数组"=w18364) -> ("十进制数值"=w18352:i32)  [unwired: 4 out]
                  }
                  frame Enabled {
                    w18370 = 255 ("高字节1")
                  }
                }
                n7207 = Build Array(w18348, w18349) -> (w18351:i32[])
              }
            }
            n7208 = Insert Into Array(array=w18282, new element=w18281) -> (w18283:dbl[])  [unwired: 1 in]
          }
          n7209 = Build Array(w18276) -> (w18275:dbl[][])
        }
        frame "温度不均衡(3)" {
          n7210 = Unbundle By Name(w18375) -> ("三级故障(从板)"=w18376:refnum<vi>)
          n7211 = property class="Clust (严格)"(reference=w18376) -> ("Value"=w18374:T8)  [unwired: 1 in, 2 out]
          n7212 = for {
            N: 7 -> [_]
            tunnel: w18374 -> [w18386]
            shift-right: [w18385] -> w18378
            shift-left: dbl[] [] -> [w18384]
            i -> [w18387]
            n7213 = case shown="5" w18387 {
              tunnel: w18386 -> [w18388 w18399 w18410 w18421 w18431 w18441 w18452]
              tunnel: [w18389 w18400 w18411 w18422 w18432 w18442 w18453] -> w18383
              frame 0, Default {
                # "电压过高"
                n7214 = disable-structure shown="启用" {
                  disable-tunnel: [w18395 w18398] -> w18391
                  disable-tunnel: [w18394 w18398] -> w18390
                  disable-tunnel: w18388 -> [w18393 _]
                  frame Disabled {
                    n7215 = Unbundle By Name(w18393) -> ("电压过高"=w18392:dbl)
                    n7216 = call "输入分辨率计算-EV05.vi"("1字节?"=FALSE, "数值"=w18392, "分辨率"=0.1) -> ("低字节"=w18394:dbl, "高字节1"=w18395:dbl)  [unwired: 2 in, 5 out]
                  }
                  frame Enabled {
                    w18398 = 255 ("高字节1")
                  }
                }
                n7217 = Build Array(w18391, w18390) -> (w18389:i32[])
              }
              frame 1 {
                # "电压过低"
                n7218 = disable-structure shown="启用" {
                  disable-tunnel: [w18406 w18409] -> w18402
                  disable-tunnel: [w18405 w18409] -> w18401
                  disable-tunnel: w18399 -> [w18404 _]
                  frame Disabled {
                    n7219 = Unbundle By Name(w18404) -> ("电压过低"=w18403:dbl)
                    n7220 = call "输入分辨率计算-EV05.vi"("1字节?"=FALSE, "数值"=w18403, "分辨率"=0.1) -> ("低字节"=w18405:dbl, "高字节1"=w18406:dbl)  [unwired: 2 in, 5 out]
                  }
                  frame Enabled {
                    w18409 = 255 ("高字节1")
                  }
                }
                n7221 = Build Array(w18402, w18401) -> (w18400:i32[])
              }
              frame 2 {
                # "电压不均衡"
                n7222 = disable-structure shown="启用" {
                  disable-tunnel: [w18417 w18420] -> w18413
                  disable-tunnel: [w18416 w18420] -> w18412
                  disable-tunnel: w18410 -> [w18415 _]
                  frame Disabled {
                    n7223 = Unbundle By Name(w18415) -> ("电压不均衡(V)"=w18414:dbl)
                    n7224 = call "输入分辨率计算-EV05.vi"("1字节?"=FALSE, "数值"=w18414, "分辨率"=0.1) -> ("低字节"=w18416:dbl, "高字节1"=w18417:dbl)  [unwired: 2 in, 5 out]
                  }
                  frame Enabled {
                    w18420 = 255 ("高字节1")
                  }
                }
                n7225 = Build Array(w18413, w18412) -> (w18411:i32[])
              }
              frame 3 {
                # "温度过高"
                n7226 = disable-structure shown="启用" {
                  disable-tunnel: [w18427 255 ("高字节1")] -> w18423
                  disable-tunnel: w18421 -> [w18425 _]
                  frame Disabled {
                    n7227 = Unbundle By Name(w18425) -> ("温度过高"=w18424:dbl)
                    n7228 = call "输入分辨率计算-EV05.vi"("1字节?"=TRUE, "数值"=w18424, "偏移量"=-40.0, "分辨率"=1.0) -> ("高字节1"=w18427:dbl)  [unwired: 1 in, 6 out]
                  }
                  frame Enabled {
                  }
                }
                n7229 = Build Array(w18423) -> (w18422:i32[])
              }
              frame 4 {
                # "温度过低"
                n7230 = disable-structure shown="启用" {
                  disable-tunnel: [w18437 255 ("高字节1")] -> w18433
                  disable-tunnel: w18431 -> [w18435 _]
                  frame Disabled {
                    n7231 = Unbundle By Name(w18435) -> ("温度过低"=w18434:dbl)
                    n7232 = call "输入分辨率计算-EV05.vi"("1字节?"=TRUE, "数值"=w18434, "偏移量"=-40.0, "分辨率"=1.0) -> ("高字节1"=w18437:dbl)  [unwired: 1 in, 6 out]
                  }
                  frame Enabled {
                  }
                }
                n7233 = Build Array(w18433) -> (w18432:i32[])
              }
              frame 5 {
                # "温度不均衡"
                n7234 = disable-structure shown="启用" {
                  disable-tunnel: [w18446 255 ("高字节1")] -> w18443
                  disable-tunnel: w18441 -> [w18445 _]
                  frame Enabled {
                    n7235 = Unbundle By Name(w18445) -> ("温度不均衡"=w18444:dbl)
                    n7236 = call "输入分辨率计算-EV05.vi"("1字节?"=TRUE, "数值"=w18444, "分辨率"=1.0) -> ("高字节1"=w18446:dbl)  [unwired: 2 in, 6 out]
                  }
                  frame Disabled {
                  }
                }
                n7237 = Build Array(w18443) -> (w18442:dbl[])
              }
              frame 6 {
                # "SOC过低"
                n7238 = disable-structure shown="启用" {
                  disable-tunnel: w18452 -> [w18469 _]
                  disable-tunnel: [w18455 w18472] -> w18451
                  disable-tunnel: [w18454 w18472] -> w18450
                  frame Disabled {
                    n7239 = Unbundle By Name(w18469) -> ("SOC过低"=w18468:dbl)
                    n7240 = call "输入分辨率计算-EV05.vi"("1字节?"=FALSE, "数值"=w18468, "分辨率"=0.1) -> ("低字节"=w18457:dbl, "高字节1"=w18458:dbl)  [unwired: 2 in, 5 out]
                    n7241 = call "二进制解析-8.6.vi"("索引"=4, "数值"=0) -> ("低位子数组"=w18461:i32[])  [unwired: 3 out]
                    n7242 = call "二进制解析-8.6.vi"("索引"=4, "数值"=w18458) -> ("低位子数组"=w18464:i32[])  [unwired: 3 out]
                    n7243 = call "二进制解析-8.6.vi"("索引"=4, "数值"=w18457) -> ("低位子数组"=w18462:i32[], "高位子数组"=w18463:i32[])  [unwired: 2 out]
                    n7244 = Insert Into Array(array=w18464, new element=w18463) -> (w18466:i32[])  [unwired: 1 in]
                    n7245 = Insert Into Array(array=w18462, new element=w18461) -> (w18460:i32[])  [unwired: 1 in]
                    n7246 = call "数值二进制转十进制-8.6.vi"("子数组"=w18460) -> ("十进制数值"=w18455:i32)  [unwired: 4 out]
                    n7247 = call "数值二进制转十进制-8.6.vi"("子数组"=w18466) -> ("十进制数值"=w18454:i32)  [unwired: 4 out]
                  }
                  frame Enabled {
                    w18472 = 255 ("高字节1")
                  }
                }
                n7248 = Build Array(w18450, w18451) -> (w18453:i32[])
              }
            }
            n7249 = Insert Into Array(array=w18384, new element=w18383) -> (w18385:dbl[])  [unwired: 1 in]
          }
          n7250 = Build Array(w18378) -> (w18377:dbl[][])
        }
        frame "SOC过低" {
          n7251 = Unbundle By Name(w18477) -> ("一级故障(从板)"=w18478:refnum<vi>)
          n7252 = property class="Clust (严格)"(reference=w18478) -> ("Value"=w18476:T8)  [unwired: 1 in, 2 out]
          n7253 = for {
            N: 7 -> [_]
            tunnel: w18476 -> [w18488]
            shift-right: [w18487] -> w18480
            shift-left: dbl[] [] -> [w18486]
            i -> [w18489]
            n7254 = case shown="6" w18489 {
              tunnel: w18488 -> [w18490 w18501 w18512 w18523 w18533 w18543 w18554]
